vi "HandleClients.vi"(8 "error in (no error)":errorcluster, 11 "S4GUI in":refnum<class "S4GUI.lvclass">) -> (0 "error out":errorcluster, 3 "S4GUI out":refnum<class "S4GUI.lvclass">)   [LabVIEW 2018, in "S4GUI.lvclass"]
uses:
  S4GUI.lvclass
  S4GUI.lvclass/S4GUI.ctl
  Publisher/Publisher.lvclass
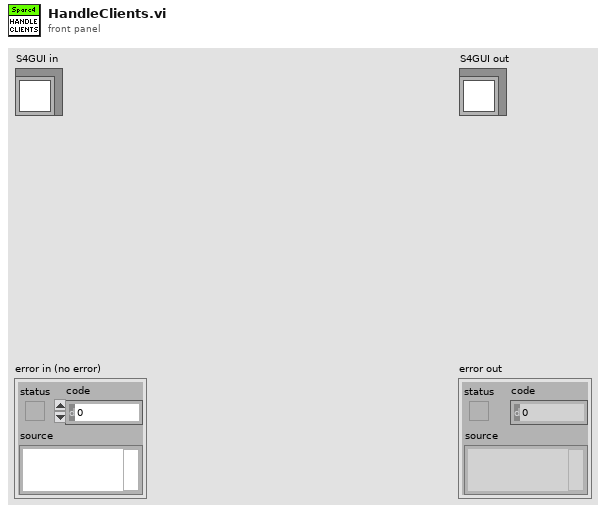
[diagram p1: front panel]
types:
  T1 = cluster{"OBSERVER":string, "OBJECT":string, "CTRLINTE":string, "PROJID":string, "SYNCMODE":string, "INSTMODE":string, "FILTER":string, "OBSTYPE":string, "CHANNEL 1":bool, "CHANNEL 2":bool, "CHANNEL 3":bool, "CHANNEL 4":bool, "TCSMODE":bool, "COMMENT":string, "broker":string, "GUIVRSN":string, "timestamp":string}
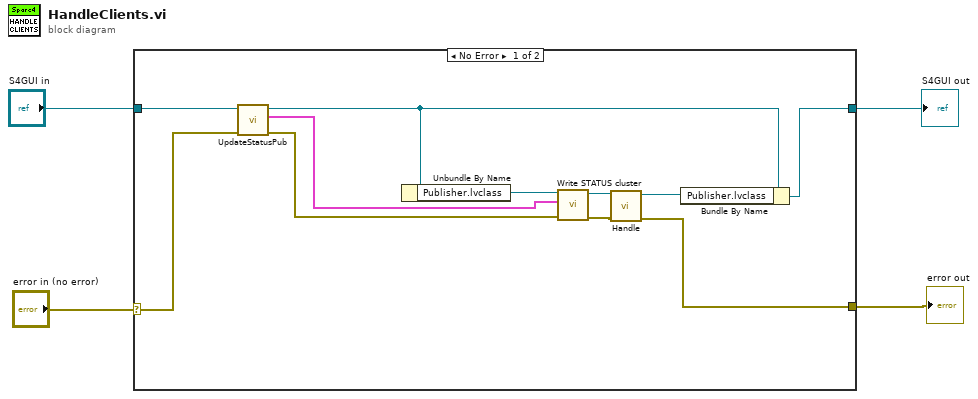
[diagram p0: block diagram]
diagram:
  n1 = case shown="No Error" "error in (no error)" {
    selector: "error in (no error)" -> [w10 w17]
    tunnel: [w6 w17] -> w3
    tunnel: [w15 w16] -> w1
    tunnel: "S4GUI in" -> [w13 w16]
    frame No Error {
      n2 = call-dynamic "UpdateStatusPub.vi"("error in (no error)"=w10, "S4GUI in"=w13) -> ("error out"=w9:errorcluster, "STATUS cluster"=w11:T1, "S4GUI out"=w12:refnum<class "S4GUI.lvclass">)  [unwired: 7 in]
      n3 = Unbundle By Name(w12) -> ("Publisher.lvclass"=w14:refnum<class "Publisher.lvclass">)
      n4 = call-dynamic "Write STATUS cluster.vi"("error in (no error)"=w9, "STATUS cluster"=w11, "Publisher in"=w14) -> ("error out"=w7:errorcluster, "Publisher out"=w8:refnum<class "Publisher.lvclass">)  [unwired: 7 in]
      n5 = call-dynamic "Handle.vi"("error in (no error)"=w7, "Publisher in"=w8) -> ("error out"=w6:errorcluster, "Publisher out"=w5:refnum<class "Publisher.lvclass">)  [unwired: 8 in]
      n6 = Bundle By Name(cluster=w12, "Publisher.lvclass"=w5) -> (w15:refnum<class "S4GUI.lvclass">)
    }
    frame Error {
    }
  }
  "error out" <- w3
  "S4GUI out" <- w1
